vi "HatchesShortBinString.vi"(6 "Units":dbl, 8 "Hatches":T1(array[cluster]), 10 "ID":u16, 11 "BinStirngIn":string) -> (3 "String":string)   [LabVIEW 2012]
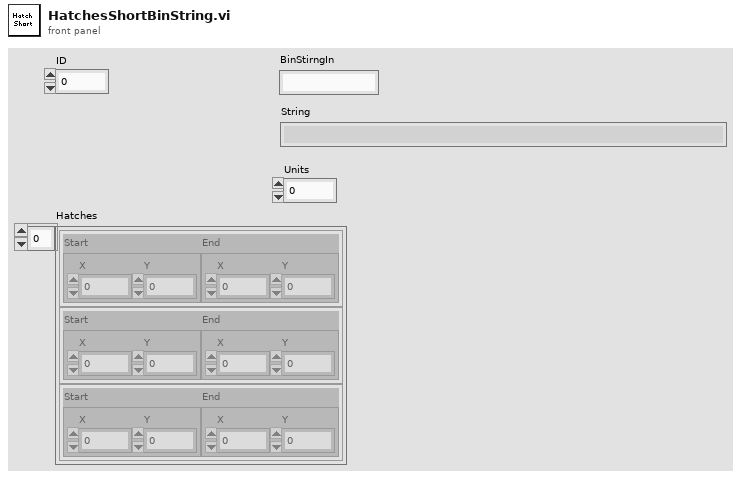
[diagram p1: front panel]
types:
  T1 = cluster{"Start":cluster{"X":dbl, "Y":dbl}, "End":cluster{"X":dbl, "Y":dbl}}[]
  T2 = enum16{"big-endian, network order", "native, host order", "little-endian"}
  T3 = cluster{"Start":cluster{"X":u16, "Y":u16}, "End":cluster{"X":u16, "Y":u16}}[]
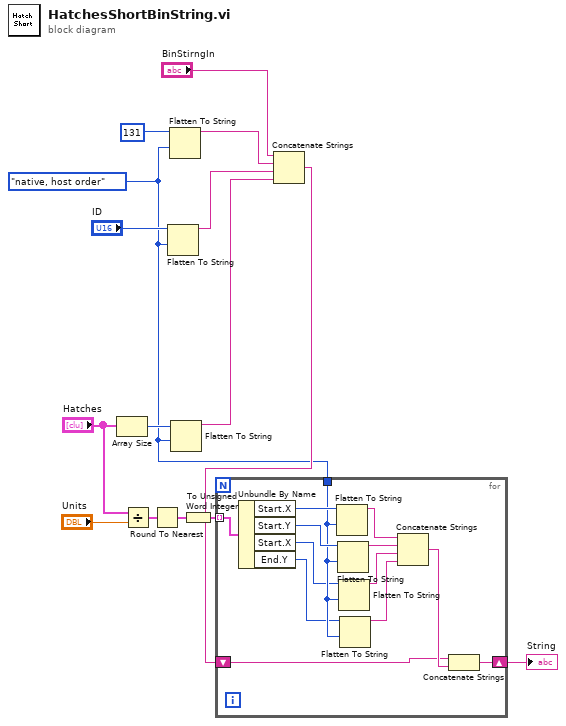
[diagram p0: block diagram]
diagram:
  w2 = T2."native, host order" ("byte order (0:big-endian, network order)")
  n1 = Array Size(array="Hatches") -> (size(s)=w13:i32)
  n2 = Divide(x="Hatches", y="Units") -> (x/y=w10:T1)
  n3 = Round To Nearest(number=w10) -> (nearest integer value=w3:T1)
  n4 = Flatten To String(anything="ID", byte order (0:big-endian, network order)=w2) -> (data string=w8:string)  [unwired: 2 in, 2 out]
  n5 = Flatten To String(anything=u16 131 ("Layer"), byte order (0:big-endian, network order)=w2) -> (data string=w9:string)  [unwired: 2 in, 2 out]
  n6 = Flatten To String(anything=w13, byte order (0:big-endian, network order)=w2) -> (data string=w7:string)  [unwired: 2 in, 2 out]
  n7 = To Unsigned Word Integer(number=w3) -> (unsigned 16bit integer=w4:T3)
  n8 = Concatenate Strings("BinStirngIn", w9, w8, w7) -> (w6:string)
  n9 = for {
    tunnel: w4 -> [w28] mode=indexing
    tunnel: w2 -> [w20]
    shift-right: [w21] -> w5
    shift-left: w6 -> [w22]
    n10 = Unbundle By Name(w28) -> ("Start.X"=w27:u16, "Start.Y"=w26:u16, "Start.X"=w19:u16, "End.Y"=w18:u16)
    n11 = Flatten To String(anything=w27, byte order (0:big-endian, network order)=w20) -> (data string=w25:string)  [unwired: 2 in, 2 out]
    n12 = Flatten To String(anything=w26, byte order (0:big-endian, network order)=w20) -> (data string=w24:string)  [unwired: 2 in, 2 out]
    n13 = Flatten To String(anything=w19, byte order (0:big-endian, network order)=w20) -> (data string=w17:string)  [unwired: 2 in, 2 out]
    n14 = Flatten To String(anything=w18, byte order (0:big-endian, network order)=w20) -> (data string=w16:string)  [unwired: 2 in, 2 out]
    n15 = Concatenate Strings(w25, w24, w17, w16) -> (w23:string)
    n16 = Concatenate Strings(w22, w23) -> (w21:string)
  }
  "String" <- w5
